vi "Run_All_LabVIEW_test_scripts.vi"() -> ()   [LabVIEW 2017]
panel:
  in  "stop":bool
  out "Status":string
  out "Total# exe :":i32
  out "# LabVIEW Test scrtipts (exe)":string
  out "Test Cases Execution Status":string
  out "#TCPass":i32
  out "#TCFail":i32
  # "- Copy this application to  \\Build\\UltraSonic_Test_Scripts and Run the application\n- This application is capable of running all the LabVIEW exe's in the Folder\n- Results will be stored in    \\Result_Next_Gen\n- Report is generated in Over_All_TC_execution_Results.txt stored @\\Result_Next_Gen"
  # "Result :"
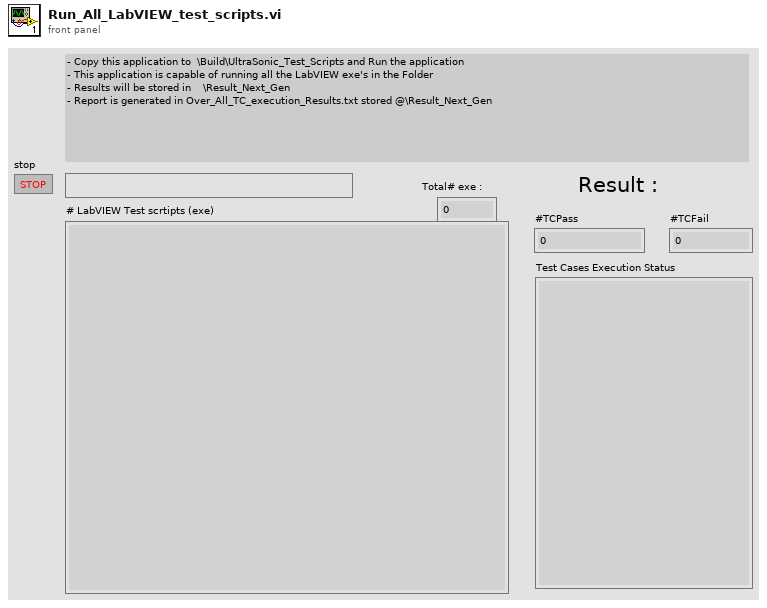
[diagram p1: front panel]
types:
  T1 = enum16{"open", "replace", "create", "open or create", "replace or create", "replace or create with confirmation"}
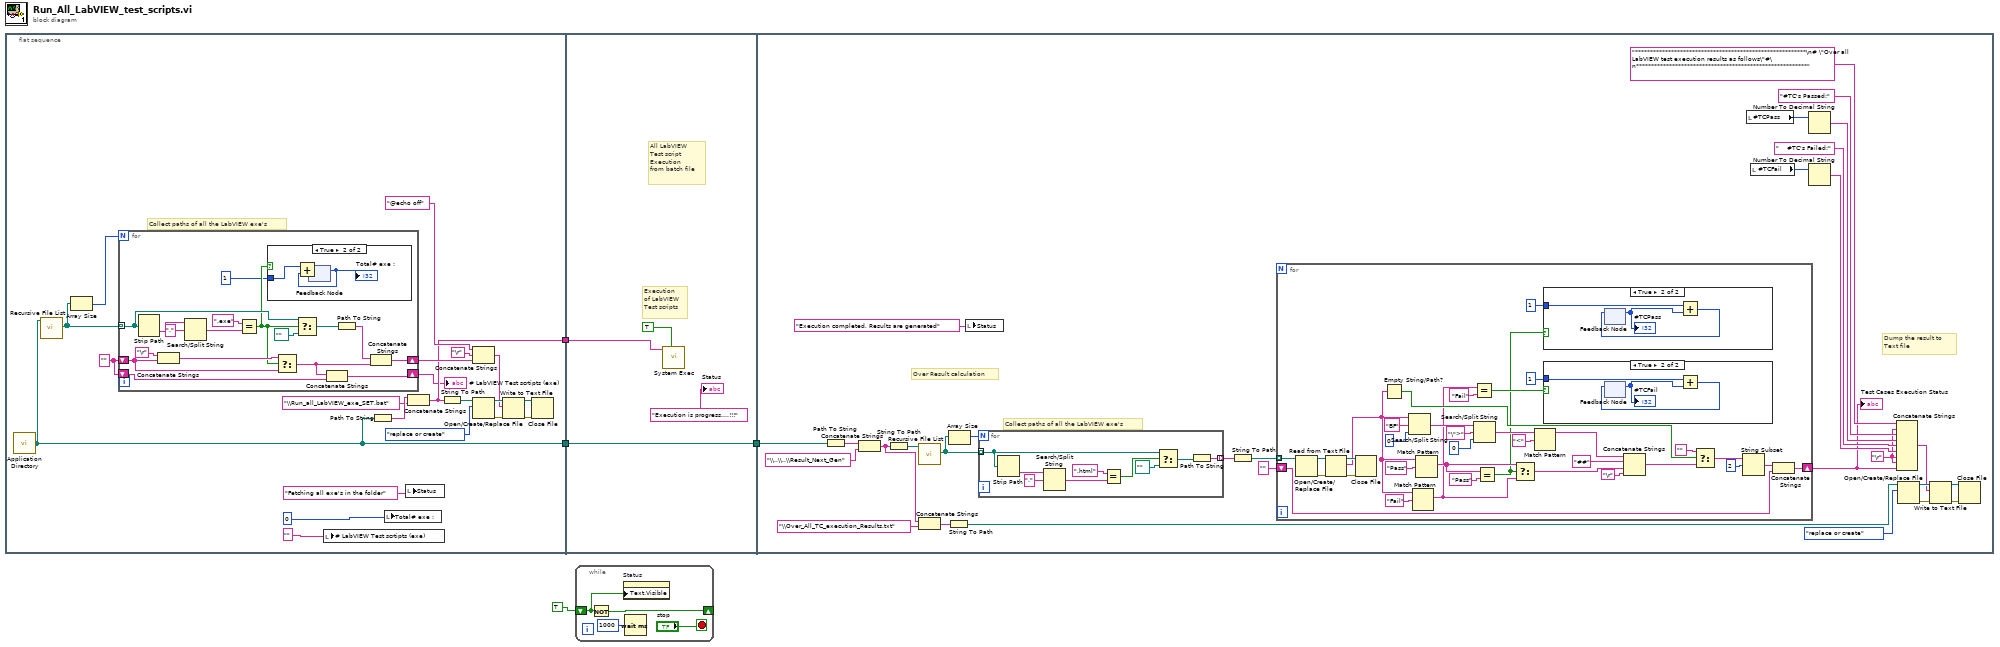
[diagram p0: block diagram]
diagram:
  n1 = flat-sequence {
    tunnel: [w11] -> w4
    tunnel: [w10] -> w2
    tunnel: w4 -> [w48]
    tunnel: [w47] -> w3
    tunnel: w2 -> [w47]
    tunnel: w3 -> [w52]
    frame #0 {
      w9 = ""
      # "Collect paths of all the LabVIEW exe's"
      n2 = call <vilib>:"Application Directory.vi"() -> ("Application Directory"=w10:path)
      n3 = call <vilib>:"Recursive File List.vi"("Folder Path"=w10) -> ("All Files in Dir"=w25:path[])  [unwired: 6 in, 4 out]
      n4 = Array Size(array=w25) -> (size(s)=w24:i32)
      n5 = for {
        N: w24 -> [_]
        tunnel: w25 -> [w38] mode=indexing
        shift-right: [w35] -> w15
        shift-left: w9 -> [w31]
        shift-right: [w29] -> w8
        shift-left: w9 -> [w28]
        n6 = Strip Path(path=w38) -> (name=w41:string)  [unwired: 1 out]
        n7 = Concatenate Strings("\r", w31) -> (w33:string)
        n8 = Search/Split String(string=w41, search string/char (-)=".") -> (match + rest of string=w40:string)  [unwired: 1 in, 2 out]
        n9 = Equal?(x=".exe", y=w40) -> (x = y?=w27:bool)
        n10 = case shown="True" w27 {
          tunnel: 1 -> [_ w45]
          frame False {
          }
          frame True {
            n11 = feedback #1() -> (w43:i32)  [unwired: 1 in]
            "Total# exe :" <- w43
            n12 = Add(x=w45, y=w43) -> (x+y=w44:i32)
            n13 = feedback-in #1(w44) -> ()
          }
        }
        n14 = Select(t=w33, s=w27, f=w31) -> (s? t:f=w30:string)
        n15 = Select(t=w38, s=w27, f=path "") -> (s? t:f=w34:path)
        n16 = Concatenate Strings(w30, w28) -> (w29:string)
        n17 = Path To String(path=w34) -> (string=w36:string)
        n18 = Concatenate Strings(w36, w30) -> (w35:string)
      }
      "# LabVIEW Test scrtipts (exe)" <- w8
      n19 = local write "# LabVIEW Test scrtipts (exe)"("" ("String")) -> ()
      n20 = Path To String(path=w10) -> (string=w14:string)
      n21 = local write "Total# exe :"(0 ("Total# exe :")) -> ()
      n22 = local write "Status"("Fetching all exe's in the folder" ("String")) -> ()
      n23 = Concatenate Strings(w14, "\\Run_all_LabVIEW_exe_SET.bat" ("string")) -> (w11:string)
      n24 = String To Path(string=w11) -> (path=w12:path)
      n25 = Concatenate Strings("@echo off" ("string"), "\r", w15) -> (w18:string)
      n26 = Open/Create/Replace File(file path (use dialog)=w12, operation (0:open)=T1."replace or create") -> (refnum out=w20:refnum<file>, error out=w23:errorcluster)  [unwired: 4 in, 1 out]
      n27 = Write to Text File(file (use dialog)=w20, text=w18, error in=w23) -> (refnum out=w22:refnum<file>, error out=w21:errorcluster)  [unwired: 1 in, 1 out]
      n28 = Close File(refnum=w22, error in=w21) -> ()  [unwired: 2 out]
    }
    frame #1 {
      # "All LabVIEW\nTest script\nExecution \nfrom batch file"
      # "Execution \nof LabVIEW\nTest scripts"
      n29 = call <vilib>:"System Exec.vi"("wait until completion? (T)"=TRUE, "command line"=w48) -> ()  [unwired: 6 in, 4 out]
      "Status" <- "Execution is progress....!!!" ("String")
    }
    frame #2 {
      w54 = "\r"
      # "Dump the result to \nText file"
      # "Over Result calculation"
      # "Collect paths of all the LabVIEW exe's"
      n30 = Path To String(path=w52) -> (string=w51:string)
      n31 = Concatenate Strings(w51, "\\..\\..\\Result_Next_Gen") -> (w58:string)
      n32 = String To Path(string=w58) -> (path=w70:path)
      n33 = call <vilib>:"Recursive File List.vi"("Folder Path"=w70) -> ("All Files in Dir"=w78:path[])  [unwired: 6 in, 4 out]
      n34 = Concatenate Strings(w58, "\\Over_All_TC_execution_Results.txt" ("string")) -> (w56:string)
      n35 = String To Path(string=w56) -> (path=w55:path)
      n36 = Array Size(array=w78) -> (size(s)=w77:i32)
      n37 = local write "Status"("Execution completed, Results are generated" ("Status")) -> ()
      n38 = for {
        N: w77 -> [_]
        tunnel: w78 -> [w124] mode=indexing
        tunnel: [w120] -> w75 mode=indexing
        n39 = Strip Path(path=w124) -> (name=w127:string)  [unwired: 1 out]
        n40 = Search/Split String(string=w127, search string/char (-)=".") -> (match + rest of string=w126:string)  [unwired: 1 in, 2 out]
        n41 = Equal?(x=".html", y=w126) -> (x = y?=w121:bool)
        n42 = Select(t=w124, s=w121, f=path "") -> (s? t:f=w122:path)
        n43 = Path To String(path=w122) -> (string=w120:string)
      }
      n44 = String To Path(string=w75) -> (path=w74:path[])
      n45 = for {
        tunnel: w74 -> [w96] mode=indexing
        shift-right: [w98] -> w53
        shift-left: "" -> [w97]
        n46 = Open/Create/Replace File(file path (use dialog)=w96) -> (refnum out=w112:refnum<file>, error out=w111:errorcluster)  [unwired: 5 in, 1 out]
        n47 = Read from Text File(file (use dialog)=w112, error in=w111) -> (refnum out=w110:refnum<file>, text=w95:string, error out=w109:errorcluster)  [unwired: 2 in, 1 out]
        n48 = Close File(refnum=w110, error in=w109) -> ()  [unwired: 2 out]
        n49 = Empty String/Path?(string/path=w95) -> (empty?=w94:bool)
        n50 = Search/Split String(string=w95, search string/char (-)="BF", offset (0)=0) -> (match + rest of string=w91:string)  [unwired: 2 out]
        n51 = Match Pattern(string=w95, regular expression="Fail") -> (match substring=w83:string)  [unwired: 1 in, 3 out]
        n52 = Match Pattern(string=w95, regular expression="Pass") -> (match substring=w102:string)  [unwired: 1 in, 3 out]
        n53 = Equal?(x=w83, y="Fail") -> (x = y?=w81:bool)
        n54 = Search/Split String(string=w91, search string/char (-)="\">" ("regular expression"), offset (0)=0) -> (match + rest of string=w90:string)  [unwired: 2 out]
        n55 = Equal?(x=w102, y="Pass") -> (x = y?=w79:bool)
        n56 = Select(t=w102, s=w79, f=w83) -> (s? t:f=w100:string)
        n57 = Match Pattern(string=w90, regular expression="<") -> (before substring=w88:string)  [unwired: 1 in, 3 out]
        n58 = case shown="True" w79 {
          tunnel: 1 -> [_ w119]
          frame False {
          }
          frame True {
            n59 = feedback #2() -> (w117:i32)  [unwired: 1 in]
            "#TCPass" <- w117
            n60 = Add(x=w119, y=w117) -> (x+y=w118:i32)
            n61 = feedback-in #2(w118) -> ()
          }
        }
        n62 = case shown="True" w81 {
          tunnel: 1 -> [_ w114]
          frame False {
          }
          frame True {
            n63 = feedback #3() -> (w115:i32)  [unwired: 1 in]
            "#TCFail" <- w115
            n64 = Add(x=w114, y=w115) -> (x+y=w116:i32)
            n65 = feedback-in #3(w116) -> ()
          }
        }
        n66 = Concatenate Strings(w88, "##" ("string"), w100, "\r") -> (w93:string)
        n67 = Select(t="", s=w94, f=w93) -> (s? t:f=w87:string)
        n68 = String Subset(string=w87, offset (0)=2) -> (substring=w85:string)  [unwired: 1 in]
        n69 = Concatenate Strings(w85, w97) -> (w98:string)
      }
      "Test Cases Execution Status" <- w53
      n70 = local read "#TCPass"() -> (w66:i32)
      n71 = local read "#TCFail"() -> (w65:i32)
      n72 = Number To Decimal String(number=w66) -> (decimal integer string=w63:string)  [unwired: 1 in]
      n73 = Number To Decimal String(number=w65) -> (decimal integer string=w61:string)  [unwired: 1 in]
      n74 = Concatenate Strings("*********************************************************\n# \"Over all LabVIEW test execution results as follows\"#\n*********************************************************" ("string"), w54, "#TC's Passed:" ("string"), w63, "    #TC's Failed:" ("string"), w61, w54, w54, w53) -> (w60:string)
      n75 = Open/Create/Replace File(file path (use dialog)=w55, operation (0:open)=T1."replace or create") -> (refnum out=w72:refnum<file>, error out=w69:errorcluster)  [unwired: 4 in, 1 out]
      n76 = Write to Text File(file (use dialog)=w72, text=w60, error in=w69) -> (refnum out=w71:refnum<file>, error out=w68:errorcluster)  [unwired: 1 in, 1 out]
      n77 = Close File(refnum=w71, error in=w68) -> ()  [unwired: 2 out]
    }
  }
  n78 = while {
    shift-right: [w131] -> _
    shift-left: TRUE -> [w132]
    stop <- "stop" stop-if-true
    n79 = Not(x=w132) -> (.not. x?=w131:bool)
    n80 = property on="Status" class="Str"("Text.Visible"=w132) -> ()  [unwired: 2 in, 2 out]
    n81 = Wait (ms)(milliseconds to wait=u32 1000) -> ()  [unwired: 1 out]
  }
